vi "Temperature RH StandAlone.vi"() -> ()   [LabVIEW 2016]
panel:
  in  "Tab Control":enum32{"Main"}(tab)
  in  "stop":bool
  in  "Scan Rate (mS)":i32=1000
  in  "Device IP Address":string="192.168.1.200"
  in  "Remote Port":u16=2000
  out "Newport ITX Data":string[][](array[string])
  in  "Open Webpage (Offsets)":bool
  # "Set Your Computer IP Address to \n(192.168.1.252). It can be any number \nbetween 2 and 254...just not 200. You might \nneed to turn off your firewall."
  # "This will work with and without Barometric Pressure\n\nThere are offsets available in the web interface. Just type\nthe 192.168.1.200 into a web browser. The default passwords\nare 00000000 and 12345678"
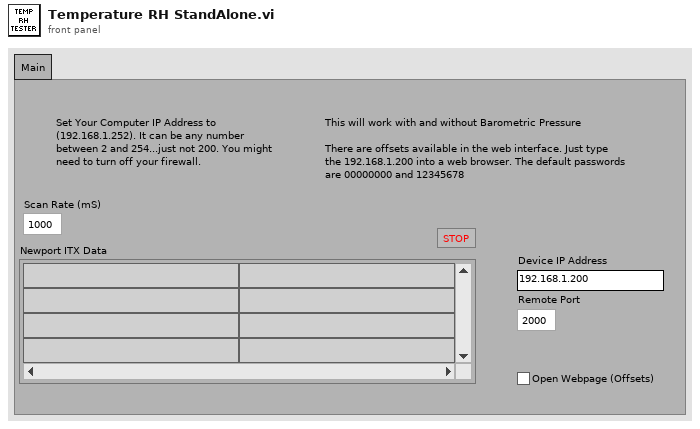
[diagram p1: front panel]
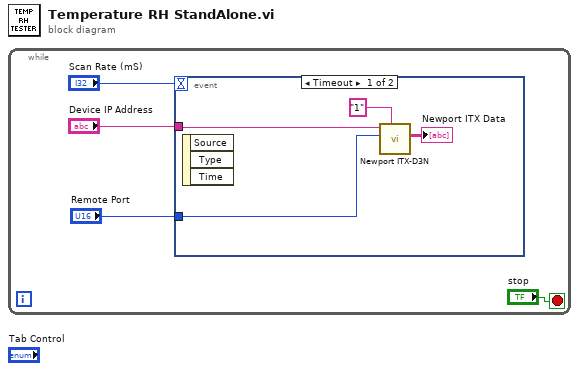
[diagram p0: block diagram]
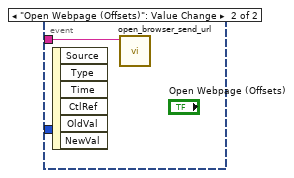
[diagram p2: hidden frame]
diagram:
  n1 = while {
    stop <- "stop" stop-if-true
    n2 = event shown="[0] Timeout" {
      selector: _ -> [_ _]
      dyn-events: _ -> [_ _]
      timeout: "Scan Rate (mS)" -> [_ _]
      tunnel: "Device IP Address" -> [w6 w9]
      tunnel: "Remote Port" -> [w5 _]
      event Timeout {
        n3 = event-data() -> ()  [unwired: 1 in, 3 out]
        n4 = call "Newport ITX-D3N.vi"("Device Number (Display In Header)"="1", "Remote Port"=w5, "Machine"=w6) -> ("Newport ITX Data"=→"Newport ITX Data":string[][])  [unwired: 5 in, 3 out]
      }
      event "Open Webpage (Offsets)": Value Change {
        n5 = event-data() -> ()  [unwired: 1 in, 6 out]
        n6 = call "open_browser_send_url.vi"("Enter a URL and run the VI"=w9) -> ()  [unwired: 11 in]
      }
    }
  }
